vi "SaveTDMS.vi"(7 "Waveform settings":T1={"Tx"=0.3, "Vx_max"=1.0, "Vy_max"=1.0, "Row_N"=20, "ratio of decline"=0.3}, 8 "错误输入（无错误）":errorcluster, 10 "数据":waveform(dbl)[](array[waveform])) -> (0 "错误输出":errorcluster)   [LabVIEW 2013]
uses:
  <vilib>/Utility/error.llb/Error Cluster From Error Code.vi
  <vilib>/ErrorRing/Error Ring.xnode
panel:
  in  "取消按钮":bool
  in  "确定按钮":bool
  in  "文件路径":path
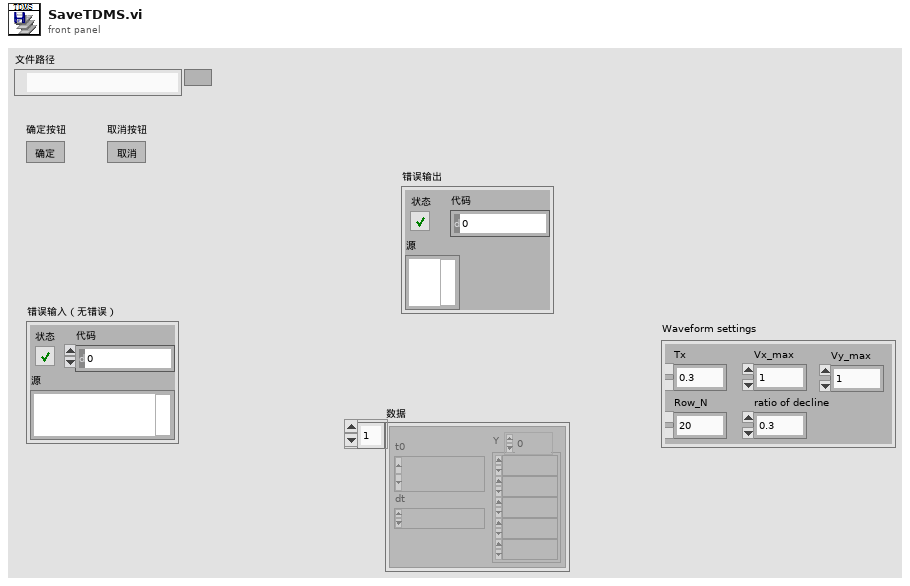
[diagram p1: front panel]
types:
  T1 = cluster{"Tx":dbl, "Vx_max":dbl, "Vy_max":dbl, "Row_N":i32, "ratio of decline":dbl}
  T2 = cluster{"Tx":dbl, "Vx_max":dbl, "Vy_max":dbl, dbl, "ratio of decline":dbl}
  T3 = enum16{"open", "open or create", "create or replace", "create", "open (read-only)"}
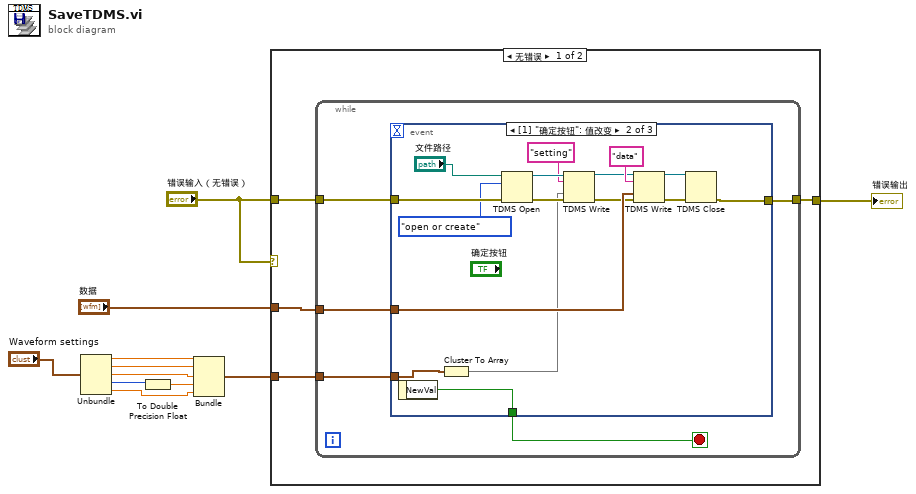
[diagram p0: block diagram]
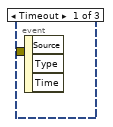
[diagram p2: hidden frame]
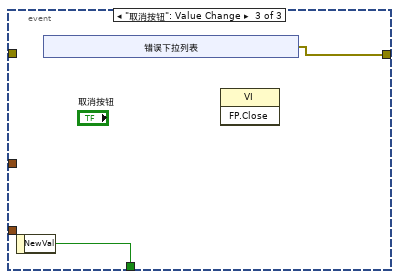
[diagram p3: hidden frame]
diagram:
  n1 = Unbundle("Waveform settings") -> ("Tx"=w3:dbl, "Vx_max"=w4:dbl, "Vy_max"=w5:dbl, "Row_N"=w6:i32, "ratio of decline"=w2:dbl)
  n2 = To Double Precision Float(number=w6) -> (double precision float=w7:dbl)
  n3 = Bundle("Tx"=w3, "Vx_max"=w4, "Vy_max"=w5, w7, "ratio of decline"=w2) -> (w1:T2)  [unwired: 1 in]
  n4 = case shown="无错误" "错误输入（无错误）" {
    tunnel: "错误输入（无错误）" -> [w15 w43]
    tunnel: [w14 w43] -> w11
    tunnel: "数据" -> [w13 _]
    tunnel: w1 -> [w12 _]
    frame No Error {
      n5 = while {
        tunnel: w13 -> [w17]
        tunnel: w15 -> [w19]
        tunnel: [w18] -> w14
        tunnel: w12 -> [w16]
        stop <- w20 stop-if-true
        n6 = event shown="[1] \"确定按钮\": 值改变" {
          selector: _ -> [_ _ _]
          dyn-events: _ -> [_ _ _]
          timeout: _ -> [_ _ _]
          tunnel: [_ w36 w38] -> w20
          tunnel: w19 -> [_ w35 _]
          tunnel: [_ w34 w37] -> w18
          tunnel: w17 -> [_ w32 _]
          tunnel: w16 -> [_ w22 _]
          event Timeout {
            n7 = event-data() -> ()  [unwired: 1 in, 3 out]
          }
          event "确定按钮": Value Change {
            n8 = event-data() -> ("NewVal"=w36:bool)  [unwired: 1 in]
            n9 = Cluster To Array(cluster=w22) -> (array=w21:dbl[])
            n10 = TDMS Open(8:w35, 10:T3."open or create" ("操作(0:open)"), 11:"文件路径") -> (0:w27:errorcluster, 3:w25:refnum<k34>)  [unwired: 4 in]
            n11 = TDMS Write(0:w25, 5:"setting" ("组名称输入（无标题）"), 9:w21, 11:w27) -> (4:w24:refnum<k34>, 15:w26:errorcluster)  [unwired: 2 in, 2 out]
            n12 = TDMS Write(0:w24, 5:"data" ("组名称输入（无标题）"), 9:w32, 11:w26) -> (4:w30:refnum<k34>, 15:w31:errorcluster)  [unwired: 2 in, 2 out]
            n13 = TDMS Close(8:w31, 11:w30) -> (0:w34:errorcluster)  [unwired: 1 out]
          }
          event "取消按钮": Value Change {
            n14 = event-data() -> ("NewVal"=w38:bool)  [unwired: 1 in]
            n15 = xnode "错误下拉列表"() -> ("错误输出"=w37:errorcluster)
            n16 = invoke class="VI" method="FP.Close"() -> ()  [unwired: 3 in, 3 out]
          }
        }
      }
    }
    frame Error {
    }
  }
  "错误输出" <- w11
